vi "FRCts20_WebMethods_Root.vi"(11 "httpRequestID":u32) -> ()   [LabVIEW 2013]
doc: "Returns the FRCts Home page.\n\nhttp://<server address>:<port>/FRCts/home"
uses:
  FRCts20_WebMethods.lvlib
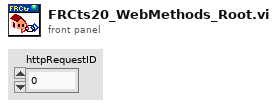
[diagram p1: front panel]
types:
  T1 = typedef "FRCts20_WebMethods.lvlib/FRCts20_WebMethods_ctl_returntype.ctl" = string
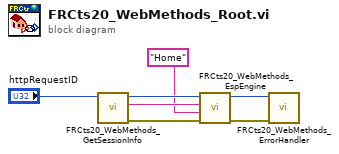
[diagram p0: block diagram]
diagram:
  n1 = call "FRCts20_WebMethods_GetSessionInfo.vi"("httpRequestID"="httpRequestID") -> ("error out"=w6:errorcluster, "Return Type"=w4:T1, "httpRequestID out"=w5:u32)  [unwired: 8 in]
  n2 = call "FRCts20_WebMethods_EspEngine.vi"("error in (no error)"=w6, "Cluster"="Home", "Return Type"=w4, "httpRequestID"=w5) -> ("error out"=w1:errorcluster, "httpRequestID out"=w7:u32)  [unwired: 6 in]
  n3 = call "FRCts20_WebMethods_ErrorHandler.vi"("error in"=w1, "httpRequestID"=w7) -> ()  [unwired: 9 in, 1 out]
